vi "Serial Configuration.vi"(8 "error in (no error)":errorcluster, 11 "FlexWorktable in":refnum<class "FlexWorktable.lvclass">) -> (0 "error out":errorcluster, 2 "Serial Configuration":T1={"timeout ms"=10000, "data bits"=8, "parity"=enum."None", "baud rate"=9600, "stop bits"=10, "flow control"=0} {"stop bits" items=["1.0"=10, "1.5"=15, "2.0"=20]; "flow control" items=["None", "XON/XOFF", "RTS/CTS", "XON/XOFF & RTS/CTS", "DTR/DSR", "XON/XOFF & DTR/DSR"]}, 3 "FlexWorktable out":refnum<class "FlexWorktable.lvclass">)   [LabVIEW 2023, in "FlexWorktable.lvclass"]
uses:
  FlexWorktable.lvclass
  FlexWorktable.lvclass/FlexWorktable.ctl
  Gantry Class/Type Definitions/Serial Configuration.ctl
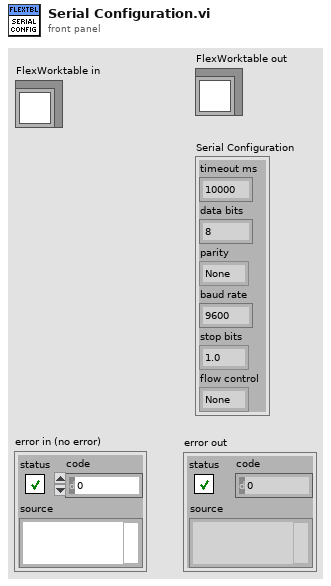
[diagram p1: front panel]
types:
  T1 = typedef "Serial Configuration.ctl" = cluster{"timeout ms":u32, "data bits":u16, "parity":enum16{"None", "Odd", "Even", "Mark", "Space"}, "baud rate":u32, "stop bits":u16, "flow control":u16}
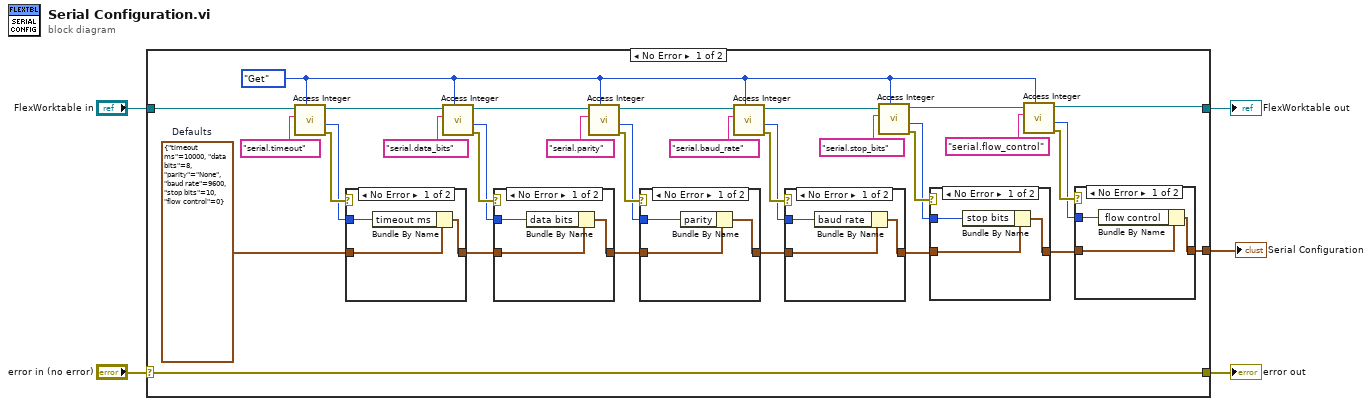
[diagram p0: block diagram]
diagram:
  n1 = case shown="No Error" "error in (no error)" {
    selector: "error in (no error)" -> [w39 w65]
    tunnel: [w39 w65] -> w4
    tunnel: [w7 w64] -> w2
    tunnel: "FlexWorktable in" -> [w38 w64]
    tunnel: [w12 _] -> w1
    frame No Error {
      w6 = enum16{"Get", "Set"}."Get" ("Get/Set")
      w35 = T1 {"timeout ms"=10000, "data bits"=8, "parity"=enum."None", "baud rate"=9600, "stop bits"=10, "flow control"=0}  # Defaults
      n2 = call-dynamic "Access Integer.vi"("Get/Set"=w6, "Key"="serial.timeout", "FlexWorktable in"=w38) -> ("error out"=w36:errorcluster, "Value out"=w34:i32, "FlexWorktable out"=w30:refnum<class "FlexWorktable.lvclass">)  [unwired: 6 in]
      n3 = case shown="No Error" w36 {
        tunnel: w35 -> [w62 w63]
        tunnel: [w61 w63] -> w29
        tunnel: w34 -> [w60 _]
        frame No Error {
          n4 = Bundle By Name(cluster=w62, "timeout ms"=w60) -> (w61:T1)
        }
        frame Error {
        }
      }
      n5 = call-dynamic "Access Integer.vi"("Get/Set"=w6, "Key"="serial.data_bits", "FlexWorktable in"=w30) -> ("error out"=w32:errorcluster, "Value out"=w31:i32, "FlexWorktable out"=w11:refnum<class "FlexWorktable.lvclass">)  [unwired: 6 in]
      n6 = case shown="No Error" w32 {
        tunnel: w29 -> [w58 w59]
        tunnel: [w57 w59] -> w16
        tunnel: w31 -> [w56 _]
        frame No Error {
          n7 = Bundle By Name(cluster=w58, "data bits"=w56) -> (w57:T1)
        }
        frame Error {
        }
      }
      n8 = call-dynamic "Access Integer.vi"("Get/Set"=w6, "Key"="serial.parity", "FlexWorktable in"=w11) -> ("error out"=w27:errorcluster, "Value out"=w26:i32, "FlexWorktable out"=w10:refnum<class "FlexWorktable.lvclass">)  [unwired: 6 in]
      n9 = case shown="No Error" w27 {
        tunnel: w16 -> [w54 w55]
        tunnel: [w53 w55] -> w15
        tunnel: w26 -> [w52 _]
        frame No Error {
          n10 = Bundle By Name(cluster=w54, "parity"=w52) -> (w53:T1)
        }
        frame Error {
        }
      }
      n11 = call-dynamic "Access Integer.vi"("Get/Set"=w6, "Key"="serial.baud_rate", "FlexWorktable in"=w10) -> ("error out"=w24:errorcluster, "Value out"=w23:i32, "FlexWorktable out"=w9:refnum<class "FlexWorktable.lvclass">)  [unwired: 6 in]
      n12 = case shown="No Error" w24 {
        tunnel: w15 -> [w50 w51]
        tunnel: [w49 w51] -> w14
        tunnel: w23 -> [w48 _]
        frame No Error {
          n13 = Bundle By Name(cluster=w50, "baud rate"=w48) -> (w49:T1)
        }
        frame Error {
        }
      }
      n14 = call-dynamic "Access Integer.vi"("Get/Set"=w6, "Key"="serial.stop_bits", "FlexWorktable in"=w9) -> ("error out"=w21:errorcluster, "Value out"=w20:i32, "FlexWorktable out"=w8:refnum<class "FlexWorktable.lvclass">)  [unwired: 6 in]
      n15 = case shown="No Error" w21 {
        tunnel: w14 -> [w46 w47]
        tunnel: [w45 w47] -> w13
        tunnel: w20 -> [w44 _]
        frame No Error {
          n16 = Bundle By Name(cluster=w46, "stop bits"=w44) -> (w45:T1)
        }
        frame Error {
        }
      }
      n17 = call-dynamic "Access Integer.vi"("Get/Set"=w6, "Key"="serial.flow_control", "FlexWorktable in"=w8) -> ("error out"=w18:errorcluster, "Value out"=w17:i32, "FlexWorktable out"=w7:refnum<class "FlexWorktable.lvclass">)  [unwired: 6 in]
      n18 = case shown="No Error" w18 {
        tunnel: w13 -> [w42 w43]
        tunnel: [w41 w43] -> w12
        tunnel: w17 -> [w40 _]
        frame No Error {
          n19 = Bundle By Name(cluster=w42, "flow control"=w40) -> (w41:T1)
        }
        frame Error {
        }
      }
    }
    frame Error {
    }
  }
  "error out" <- w4
  "FlexWorktable out" <- w2
  "Serial Configuration" <- w1
